vi "tm430_functions_41.vi"() -> ()   [LabVIEW 2011]
panel:
  in  "View":dbl min=0.0 max=2.0 step=1.0
  out "Image":u16[][](graph)
  in  "Snap":bool
  in  "Parameter":u32(ring)=4212128 items=["SENSOR MODE"=4212128, "READOUT SPEED"=4211872, "READOUT DIRECTION"=4211904, "TRIGGER GLOBAL EXPOSURE"=2049680, "TRIGGER DELAY"=1066480, "INTERNAL TRIGGER HANDLING"=1066496, "SENSOR TEMPERATURE"=2115232, "SENSOR COOLER STATUS"=2115280, "EXPOSURE TIME"=2049184, "DEFECT CORRECT MODE"=4670368, "HOT PIXEL CORRECT LEVEL"=4670400, "BINNING"=4215968, "INTERNAL LINE SPEED"=4226000, "INTERNAL LINE INTERVAL"=4226016, "IMAGE PIXEL TYPE"=4343296, "NUMBER OF OUTPUT TRIGGER CONNECTOR"=1852320, "OUTPUT TRIGGER SOURCE[0]"=1852576, "OUTPUT TRIGGER SOURCE[1]"=1852832, "OUTPUT TRIGGER SOURCE[2]"=1853088, "OUTPUT TRIGGER POLARITY[0]"=1852592, "OUTPUT TRIGGER POLARITY[1]"=1852848, "OUTPUT TRIGGER POLARITY[2]"=1853104, "OUTPUT TRIGGER ACTIVE[0]"=1852608, "OUTPUT TRIGGER ACTIVE[1]"=1852864, "OUTPUT TRIGGER ACTIVE[2]"=1853120, "OUTPUT TRIGGER DELAY[0]"=1852624, "OUTPUT TRIGGER DELAY[1]"=1852880, "OUTPUT TRIGGER DELAY[2]"=1853136, "OUTPUT TRIGGER PERIOD[0]"=1852640, "OUTPUT TRIGGER PERIOD[1]"=1852896, "OUTPUT TRIGGER PERIOD[2]"=1853152, "OUTPUT TRIGGER KIND[0]"=1852656, "OUTPUT TRIGGER KIND[1]"=1852912, "OUTPUT TRIGGER KIND[2]"=1853168, "OUTPUT TRIGGER BASE SENSOR[0]"=1852672, "OUTPUT TRIGGER BASE SENSOR[1]"=1852928, "OUTPUT TRIGGER BASE SENSOR[2]"=1853184, "OUTPUT TRIGGER PRE HSYNC COUNT"=1852704]
  in  "Text Value":dbl(ring) items=["FORWARD"=1.0, "BACKWARD"=2.0]
  in  "Value":dbl(slide) min=1.0 max=2.0 scale=1.0..2.0
  out "error out":errorcluster
  in  "stop":bool
  # "This example shows a way you can access\nmany of the functions available to the camera and see how they affect the captured image."
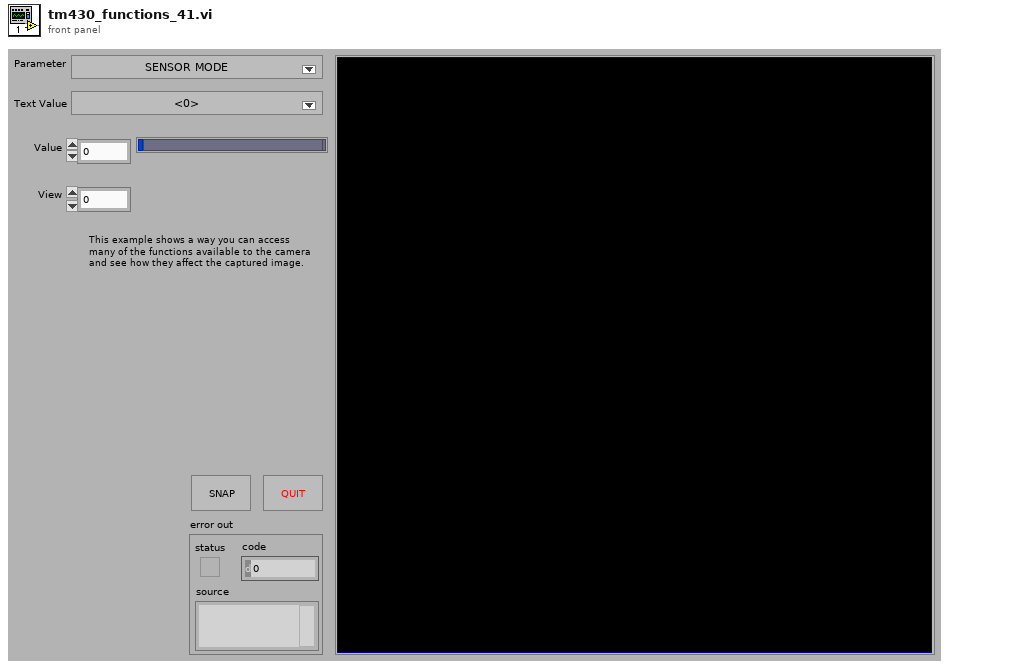
[diagram p1: front panel]
types:
  T1 = enum8{"Enabled", "Disabled", "Disabled and Grayed Out"}
  T2 = cluster{"Function Name":string, "Function ID":u32}[]
  T3 = cluster{"Function Name":string, "Function ID":u32}
  T4 = cluster{"Range":cluster{"min":dbl, "max":dbl, "step":dbl}, "default":dbl, "views":u32, "Writable":bool, "Text Values":bool, "Value Names":cluster{"Name":string, "Value":dbl}[]}
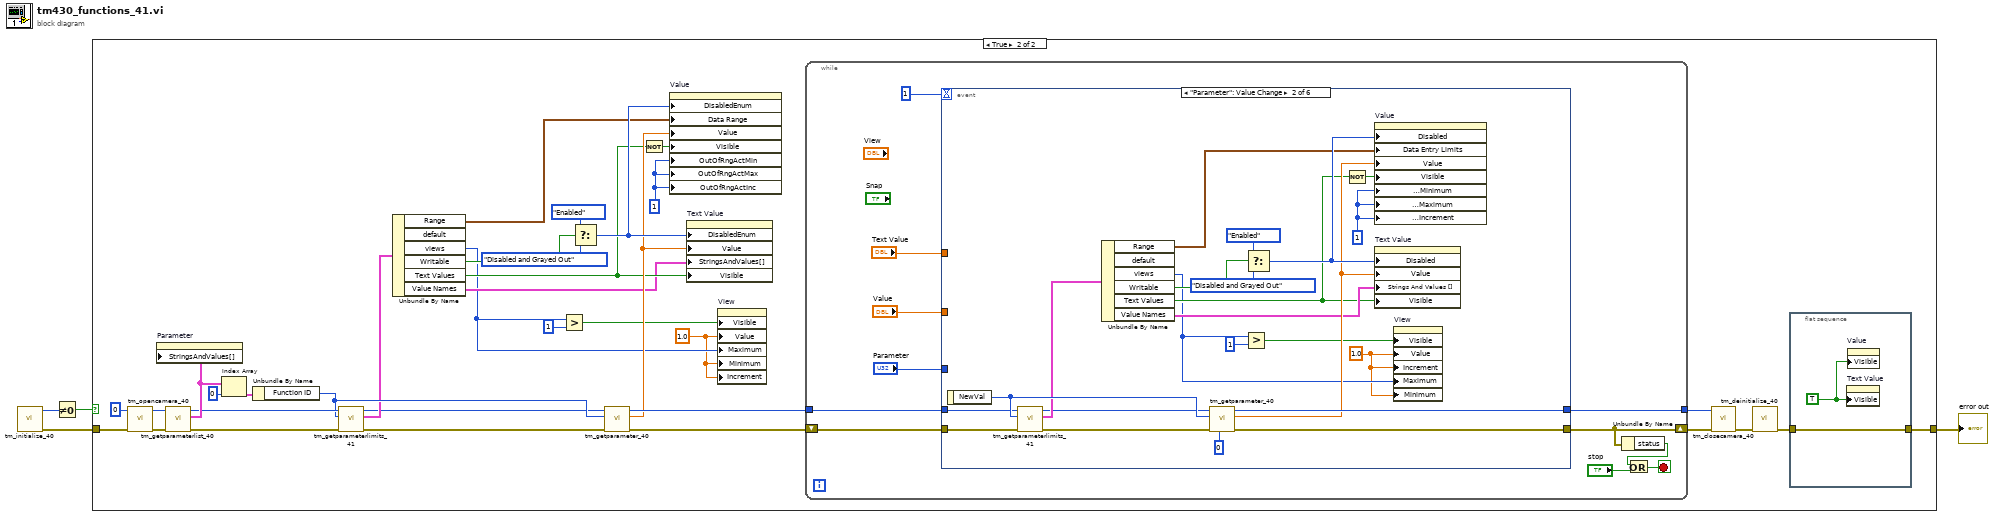
[diagram p0: block diagram]
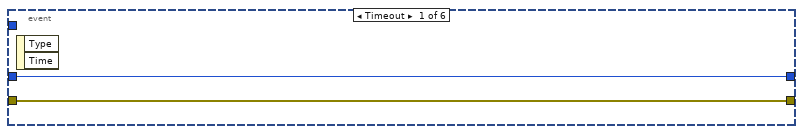
[diagram p3: hidden frame]
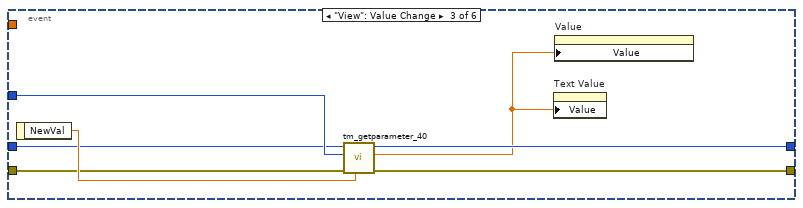
[diagram p4: hidden frame]
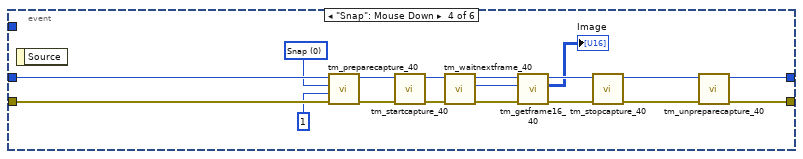
[diagram p5: hidden frame]
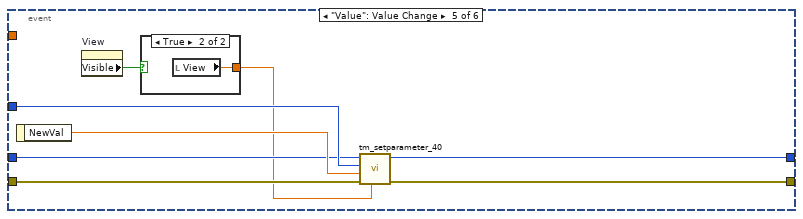
[diagram p6: hidden frame]
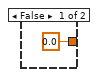
[diagram p7: hidden frame]
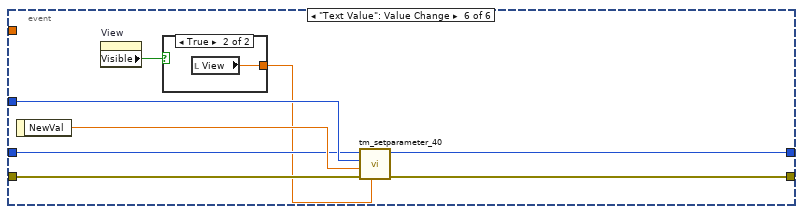
[diagram p8: hidden frame]
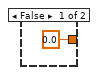
[diagram p9: hidden frame]
diagram:
  n1 = call <userlib>:"tm_initialize_40.vi"() -> ("error out"=w2:errorcluster, "Number Of Cameras"=w4:u32)  [unwired: 8 in, 2 out]
  n2 = Not Equal To 0?(x=w4) -> (x != 0?=w3:bool)
  n3 = case shown="True" w3 {
    tunnel: [w5 w34] -> w1
    tunnel: w2 -> [w5 w39]
    frame False {
    }
    frame True {
      w6 = 1.0 ("View")
      w26 = u8 1 ("Out Of Range Action:Increment")
      n4 = call <userlib>:"tm_opencamera_40.vi"("error in (no error)"=w39, "Camera Index"=u32 0) -> ("error out"=w36:errorcluster, "Handle out"=w37:u32)  [unwired: 7 in, 1 out]
      n5 = call <userlib>:"tm_getparameterlist_40.vi"("error in (no error)"=w36, "Handle in"=w37) -> ("error out"=w17:errorcluster, "Function List"=w22:T2, "Handle out"=w19:u32)  [unwired: 7 in]
      n6 = property on="Parameter" class="Ring (strict)"("StringsAndValues[]"=w22) -> ()  [unwired: 2 in, 2 out]
      n7 = Index Array(array=w22, index=0) -> (element=w20:T3)
      n8 = Unbundle By Name(w20) -> ("Function ID"=w18:u32)
      n9 = call <userlib>:"tm_getparameterlimits_41.vi"("error in (no error)"=w17, "Parameter"=w18, "Handle in"=w19) -> ("error out"=w11:errorcluster, "Limits"=w16:T4, "Handle out"=w10:u32)  [unwired: 6 in]
      n10 = Unbundle By Name(w16) -> ("Range"=w15:cluster{"min":dbl, "max":dbl, "step":dbl}, "views"=w7:u32, "Writable"=w14:bool, "Text Values"=w13:bool, "Value Names"=w12:cluster{"Name":string, "Value":dbl}[])  [unwired: 1 out]
      n11 = Greater?(x=w7, y=u32 1) -> (0:w8:bool)
      n12 = Select(t=T1."Enabled" ("Disabled"), s=w14, f=T1."Disabled and Grayed Out" ("Disabled")) -> (s? t:f=w28:T1)
      n13 = call <userlib>:"tm_getparameter_40.vi"("error in (no error)"=w11, "Parameter"=w18, "Handle in"=w10) -> ("error out"=w23:errorcluster, "Value out"=w24:dbl, "Handle out"=w25:u32)  [unwired: 6 in]
      n14 = Not(x=w13) -> (.not. x?=w27:bool)
      n15 = property on="Value" class="Slide (strict)"("DisabledEnum"=w28, "Data Range"=w15, "Value"=w24, "Visible"=w27, "OutOfRngActMin"=w26, "OutOfRngActMax"=w26, "OutOfRngActInc"=w26) -> ()  [unwired: 2 in, 2 out]
      n16 = property on="Text Value" class="Ring (strict)"("DisabledEnum"=w28, "Value"=w24, "StringsAndValues[]"=w12, "Visible"=w13) -> ()  [unwired: 2 in, 2 out]
      n17 = property on="View" class="DigNum (strict)"("Visible"=w8, "Value"=w6, "Maximum"=w7, "Minimum"=w6, "Increment"=w6) -> ()  [unwired: 2 in, 2 out]
      n18 = while {
        tunnel: w25 -> [w48]
        tunnel: [w46] -> w32
        shift-right: [w45] -> w33
        shift-left: w23 -> [w49]
        stop <- w50 stop-if-true
        n19 = event shown="[1] \"Parameter\": Value Change" {
          selector: _ -> [_ _ _ _ _ _]
          dyn-events: _ -> [_ _ _ _ _ _]
          timeout: 1 -> [_ _ _ _ _ _]
          tunnel: w49 -> [w54 w67 w78 w101 w110 w120]
          tunnel: w48 -> [w53 w68 w79 w102 w107 w116]
          tunnel: [w53 w72 w84 w92 w106 w115] -> w46
          tunnel: [w54 w70 w82 w91 w105 w119] -> w45
          tunnel: "Parameter" -> [_ _ w81 _ w108 w117]
          tunnel: "Value" -> [_ _ _ _ _ _]
          tunnel: "Text Value" -> [_ _ _ _ _ _]
          event Timeout {
            n20 = event-data() -> ()  [unwired: 1 in, 2 out]
          }
          event "Parameter": Value Change {
            w55 = 1.0 ("View")
            w76 = u8 1 ("Out Of Range Action:Increment")
            n21 = event-data() -> ("NewVal"=w69:u32)  [unwired: 1 in]
            n22 = call <userlib>:"tm_getparameterlimits_41.vi"("error in (no error)"=w67, "Parameter"=w69, "Handle in"=w68) -> ("error out"=w64:errorcluster, "Limits"=w66:T4, "Handle out"=w65:u32)  [unwired: 6 in]
            n23 = Unbundle By Name(w66) -> ("Range"=w63:cluster{"min":dbl, "max":dbl, "step":dbl}, "views"=w56:u32, "Writable"=w62:bool, "Text Values"=w60:bool, "Value Names"=w61:cluster{"Name":string, "Value":dbl}[])  [unwired: 1 out]
            n24 = call <userlib>:"tm_getparameter_40.vi"("Index"=0, "error in (no error)"=w64, "Parameter"=w69, "Handle in"=w65) -> ("error out"=w70:errorcluster, "Value out"=w71:dbl, "Handle out"=w72:u32)  [unwired: 5 in]
            n25 = Greater?(x=w56, y=u32 1) -> (0:w58:bool)
            n26 = Select(t=T1."Enabled" ("Disabled"), s=w62, f=T1."Disabled and Grayed Out" ("Disabled")) -> (s? t:f=w75:T1)
            n27 = Not(x=w60) -> (.not. x?=w77:bool)
            n28 = property on="Value" class="Slide (strict)"("Disabled"=w75, "Data Entry Limits"=w63, "Value"=w71, "Visible"=w77, "Response to Value Outside Limits:Minimum"=w76, "Response to Value Outside Limits:Maximum"=w76, "Response to Value Outside Limits:Increment"=w76) -> ()  [unwired: 2 in, 2 out]
            n29 = property on="Text Value" class="Ring (strict)"("Disabled"=w75, "Value"=w71, "Strings And Values []"=w61, "Visible"=w60) -> ()  [unwired: 2 in, 2 out]
            n30 = property on="View" class="DigNum (strict)"("Visible"=w58, "Value"=w55, "Increment"=w55, "Maximum"=w56, "Minimum"=w55) -> ()  [unwired: 2 in, 2 out]
          }
          event "View": Value Change {
            n31 = event-data() -> ("NewVal"=w80:dbl)  [unwired: 1 in]
            n32 = call <userlib>:"tm_getparameter_40.vi"("Index"=w80, "error in (no error)"=w78, "Parameter"=w81, "Handle in"=w79) -> ("error out"=w82:errorcluster, "Value out"=w83:dbl, "Handle out"=w84:u32)  [unwired: 5 in]
            n33 = property on="Text Value" class="Ring (strict)"("Value"=w83) -> ()  [unwired: 2 in, 2 out]
            n34 = property on="Value" class="Slide (strict)"("Value"=w83) -> ()  [unwired: 2 in, 2 out]
          }
          event "Snap": Mouse Down {
            w100 = 0 items=["Snap", "Sequence"] ("Capture mode")
            n35 = event-data() -> ()  [unwired: 1 in, 1 out]
            n36 = call <userlib>:"tm_preparecapture_40.vi"("error in (no error)"=w101, "Frames"=1, "Capture mode"=w100, "Handle in"=w102) -> ("error out"=w98:errorcluster, "Handle out"=w97:u32)  [unwired: 4 in, 2 out]
            n37 = call <userlib>:"tm_startcapture_40.vi"("error in (no error)"=w98, "Handle in"=w97) -> ("error out"=w89:errorcluster, "Handle out"=w90:u32)  [unwired: 8 in]
            n38 = call <userlib>:"tm_waitnextframe_40.vi"("error in (no error)"=w89, "Handle in"=w90) -> ("error out"=w87:errorcluster, "Frame Index"=w85:i32, "Handle out"=w88:u32)  [unwired: 6 in, 1 out]
            n39 = call <userlib>:"tm_getframe16_40.vi"("error in (no error)"=w87, "Frame Index"=w85, "Handle in"=w88) -> ("error out"=w95:errorcluster, "Data"=→"Image":u16[][], "Handle out"=w96:u32)  [unwired: 5 in, 1 out]
            n40 = call <userlib>:"tm_stopcapture_40.vi"("error in (no error)"=w95, "Handle in"=w96) -> ("error out"=w94:errorcluster, "Handle out"=w93:u32)  [unwired: 8 in]
            n41 = call <userlib>:"tm_unpreparecapture_40.vi"("error in (no error)"=w94, "Handle in"=w93) -> ("error out"=w91:errorcluster, "Handle out"=w92:u32)  [unwired: 8 in]
          }
          event "Value": Value Change {
            n42 = event-data() -> ("NewVal"=w109:dbl)  [unwired: 1 in]
            n43 = property on="View" class="DigNum (strict)"() -> ("Visible"=w104:bool)  [unwired: 2 in, 2 out]
            n44 = case shown="True" w104 {
              tunnel: [0.0 ("View") w112] -> w103
              frame False {
              }
              frame True {
                n45 = local read "View"() -> (w112:dbl)
              }
            }
            n46 = call <userlib>:"tm_setparameter_40.vi"("Index"=w103, "error in (no error)"=w110, "Value in"=w109, "Parameter"=w108, "Handle in"=w107) -> ("error out"=w105:errorcluster, "Handle out"=w106:u32)  [unwired: 5 in]
          }
          event "Text Value": Value Change {
            n47 = event-data() -> ("NewVal"=w118:dbl)  [unwired: 1 in]
            n48 = property on="View" class="DigNum (strict)"() -> ("Visible"=w114:bool)  [unwired: 2 in, 2 out]
            n49 = case shown="True" w114 {
              tunnel: [0.0 ("View") w122] -> w113
              frame False {
              }
              frame True {
                n50 = local read "View"() -> (w122:dbl)
              }
            }
            n51 = call <userlib>:"tm_setparameter_40.vi"("Index"=w113, "error in (no error)"=w120, "Value in"=w118, "Parameter"=w117, "Handle in"=w116) -> ("error out"=w119:errorcluster, "Handle out"=w115:u32)  [unwired: 5 in]
          }
        }
        n52 = Unbundle By Name(w45) -> ("status"=w51:bool)
        n53 = Or(x=w51, y="stop") -> (x .or. y?=w50:bool)
      }
      n54 = call <userlib>:"tm_closecamera_40.vi"("error in (no error)"=w33, "Handle in"=w32) -> ("error out"=w38:errorcluster)  [unwired: 9 in]
      n55 = call <userlib>:"tm_deinitialize_40.vi"("error in (no error)"=w38) -> ("error out"=w35:errorcluster)  [unwired: 10 in]
      n56 = flat-sequence {
        tunnel: w35 -> [w41]
        tunnel: [w41] -> w34
        frame #0 {
          w40 = TRUE
          n57 = property on="Text Value" class="Ring (strict)"("Visible"=w40) -> ()  [unwired: 2 in, 2 out]
          n58 = property on="Value" class="Slide (strict)"("Visible"=w40) -> ()  [unwired: 2 in, 2 out]
        }
      }
    }
  }
  "error out" <- w1
